vi "GPS Serial Talk.vi"(8 "error in (no error)":errorcluster, 10 "Input buffer refnum":refnum<vi>, 11 "VISAResourceName in":refnum<vi>) -> (0 "error out":errorcluster)   [LabVIEW 2016]
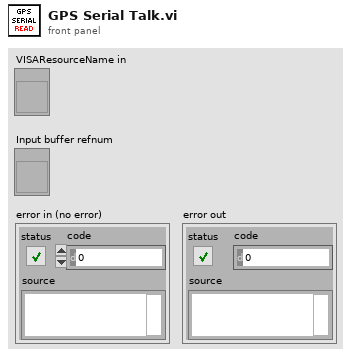
[diagram p1: front panel]
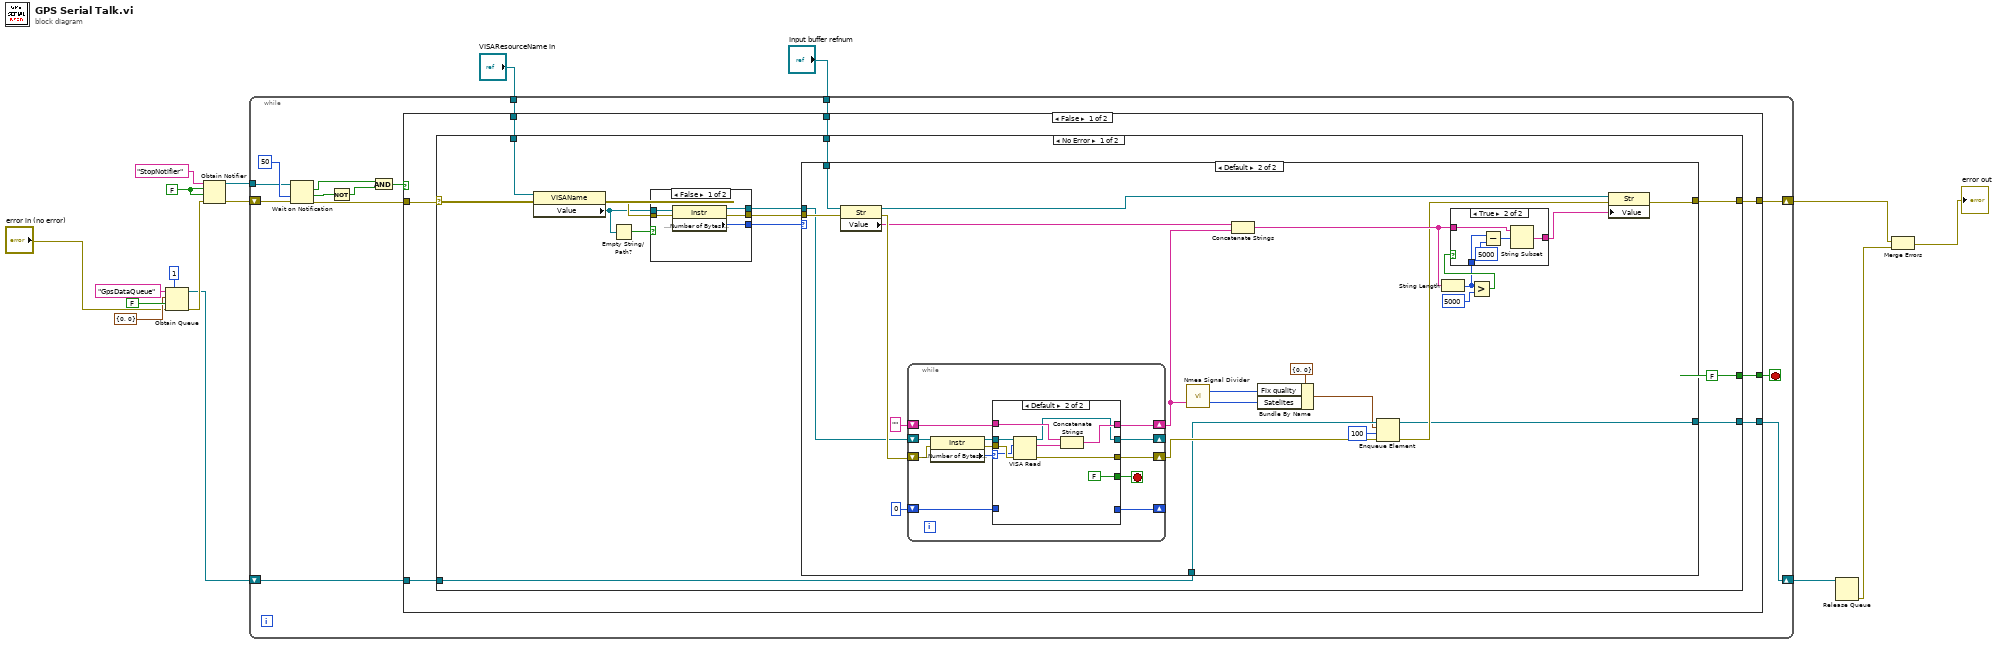
[diagram p0: block diagram]
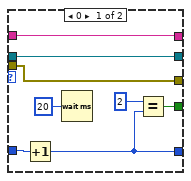
[diagram p4: hidden frame]
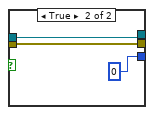
[diagram p5: hidden frame]
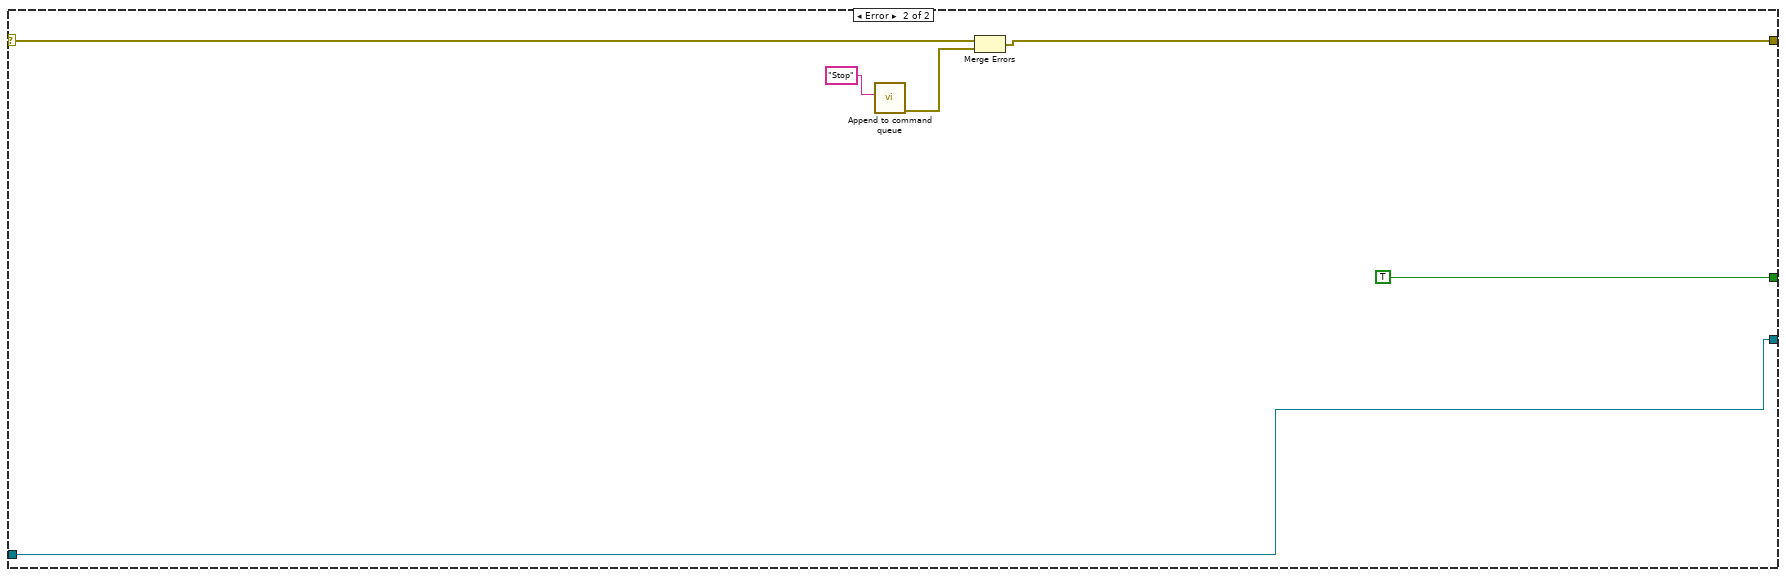
[diagram p6: hidden frame]
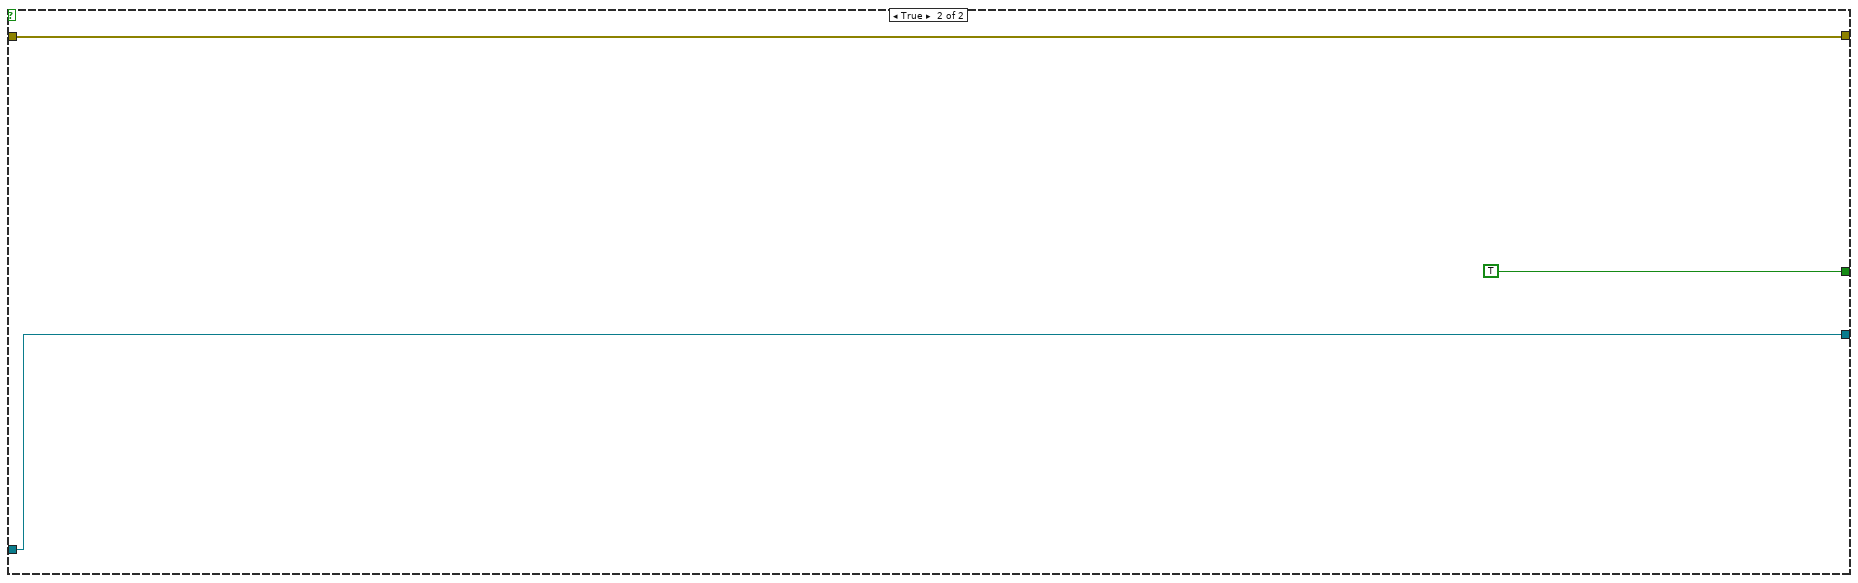
[diagram p7: hidden frame]
diagram:
  w17 = FALSE
  n1 = Obtain Queue(max queue size (-1, unlimited)=1, name (unnamed)="GpsDataQueue", element data type=cluster{"Fix quality":i8, "Satelites":i8} {"Fix quality"=0, "Satelites"=0}, create if not found? (T)=FALSE, error in (no error)="error in (no error)") -> (queue out=w5:refnum<queue>, error out=w7:errorcluster)  [unwired: 1 out]
  n2 = Obtain Notifier(name (unnamed)="StopNotifier", notification data type=w17, create if not found? (T)=w17, error in (no error)=w7) -> (notifier out=w15:refnum<notifier>, error out=w14:errorcluster)  [unwired: 1 out]
  n3 = while {
    shift-right: [w31] -> w2
    shift-left: w14 -> [w29]
    tunnel: w15 -> [w22]
    tunnel: "Input buffer refnum" -> [w21]
    tunnel: "VISAResourceName in" -> [w20]
    shift-right: [w18] -> w4
    shift-left: w5 -> [w19]
    stop <- w23 stop-if-true
    n4 = Wait on Notification(notifier=w22, timeout in ms (-1)=u32 50 ("milliseconds to wait"), error in (no error)=w29) -> (notification=w26:bool, timed out?=w28:bool, error out=w24:errorcluster)  [unwired: 1 in, 1 out]
    n5 = Not(x=w28) -> (.not. x?=w27:bool)
    n6 = And(x=w26, y=w27) -> (x .and. y?=w25:bool)
    n7 = case shown="False" w25 {
      tunnel: [w38 w128] -> w31
      tunnel: w24 -> [w37 w128]
      tunnel: [w36 TRUE] -> w23
      tunnel: w21 -> [w35 _]
      tunnel: w20 -> [w34 _]
      tunnel: w19 -> [w33 w127]
      tunnel: [w32 w127] -> w18
      frame False {
        n8 = case shown="No Error" w37 {
          selector: w37 -> [w46 w125]
          tunnel: [w47 w124] -> w38
          tunnel: [FALSE TRUE] -> w36
          tunnel: w35 -> [w42 _]
          tunnel: w34 -> [w41 _]
          tunnel: w33 -> [w40 w121]
          tunnel: [w39 w121] -> w32
          frame No Error {
            n9 = property on="Property Node" class="VISAName"(reference=w41, error in=w46) -> (error out=w51:errorcluster, "Value"=w44:refnum<visa-resource-name>)  [unwired: 1 out]
            n10 = Empty String/Path?(string/path=w44) -> (empty?=w43:bool)
            n11 = case shown="False" w43 {
              tunnel: w51 -> [w117 w119]
              tunnel: [w116 u32 0 ("Bytes at Port")] -> w50
              tunnel: [w115 w118] -> w49
              tunnel: [w114 w119] -> w48
              tunnel: w44 -> [w113 w118]
              frame False {
                n12 = property class="Instr"(reference=w113, error in=w117) -> (reference out=w115:refnum<visa-resource-name>, error out=w114:errorcluster, "Serial Settings:Number of Bytes at Serial Port"=w116:u32)
              }
              frame True {
              }
            }
            n13 = case shown="Default" w50 {
              tunnel: w49 -> [_ w73]
              tunnel: w48 -> [w53 w76]
              tunnel: [w53 w77] -> w47
              tunnel: w42 -> [_ w65]
              tunnel: w40 -> [w52 w60]
              tunnel: [w52 w54] -> w39
              frame 0 {
              }
              frame Default {
                n14 = property on="Property Node" class="Str"(reference=w65, error in=w76) -> (reference out=w75:refnum<vi>, error out=w74:errorcluster, "Value"=w66:string)
                n15 = while {
                  shift-right: [w92] -> w63
                  shift-left: "" -> [w93]
                  shift-right: [w89] -> w62
                  shift-left: w74 -> [w88]
                  shift-right: [w85] -> _
                  shift-left: 0 -> [w86]
                  shift-right: [w84] -> _
                  shift-left: w73 -> [w87]
                  stop <- w94 stop-if-true
                  n16 = property class="Instr"(reference=w87, error in=w88) -> (reference out=w91:refnum<visa-resource-name>, error out=w90:errorcluster, "Serial Settings:Number of Bytes at Serial Port"=w95:u32)
                  n17 = case shown="Default" w95 {
                    selector: w95 -> [_ w106]
                    tunnel: [w99 FALSE] -> w94
                    tunnel: w93 -> [w103 w110]
                    tunnel: [w103 w111] -> w92
                    tunnel: w91 -> [w96 w112]
                    tunnel: w90 -> [w102 w107]
                    tunnel: [w102 w105] -> w89
                    tunnel: w86 -> [w100 _]
                    tunnel: [w98 _] -> w85
                    tunnel: [w96 w104] -> w84
                    frame 0 {
                      n18 = Increment(x=w100) -> (x+1=w98:i32)
                      n19 = Wait (ms)(milliseconds to wait=u32 20) -> ()  [unwired: 1 out]
                      n20 = Equal?(x=2, y=w98) -> (x = y?=w99:bool)
                    }
                    frame Default {
                      n21 = VISA Read(VISA resource name=w112, byte count=w106, error in (no error)=w107) -> (VISA resource name out=w104:refnum<visa-resource-name>, read buffer=w109:string, error out=w105:errorcluster)  [unwired: 1 out]
                      n22 = Concatenate Strings(w110, w109) -> (w111:string)
                    }
                  }
                }
                n23 = call "Nmea Signal Divider.vi"("NMEA in"=w63) -> ("Satelites"=w57:i8, "Fix quality"=w56:i8)  [unwired: 1 in]
                n24 = Concatenate Strings(w66, w63) -> (w64:string)
                n25 = Bundle By Name(cluster=cluster{"Fix quality":i8, "Satelites":i8} {"Fix quality"=0, "Satelites"=0} ("element"), "Fix quality"=w56, "Satelites"=w57) -> (w55:cluster{"Fix quality":i8, "Satelites":i8})
                n26 = Enqueue Element(queue=w60, element=w55, timeout in ms (-1)=100, error in (no error)=w62) -> (queue out=w54:refnum<queue>, error out=w61:errorcluster)  [unwired: 1 out]
                n27 = String Length(string=w64) -> (length=w68:i32)
                n28 = Greater?(x=w68, y=5000) -> (0:w69:bool)
                n29 = case shown="True" w69 {
                  tunnel: w68 -> [_ w83]
                  tunnel: w64 -> [w78 w80]
                  tunnel: [w78 w79] -> w67
                  frame False {
                  }
                  frame True {
                    n30 = Subtract(x=w83, y=5000) -> (x-y=w81:i32)
                    n31 = String Subset(string=w80, offset (0)=w81) -> (substring=w79:string)  [unwired: 1 in]
                  }
                }
                n32 = property on="Property Node" class="Str"(reference=w75, error in=w61, "Value"=w67) -> (error out=w77:errorcluster)  [unwired: 1 out]
              }
            }
          }
          frame Error {
            n33 = call "Append to command queue.vi"("Single command"="Stop") -> ("error out"=w123:errorcluster)  [unwired: 10 in]
            n34 = Merge Errors(w125, w123) -> (w124:errorcluster)
          }
        }
      }
      frame True {
      }
    }
  }
  n35 = Release Queue(queue=w4) -> (error out=w1:errorcluster)  [unwired: 2 in, 2 out]
  n36 = Merge Errors(w2, w1) -> (→"error out":errorcluster)
